vi "Build Menu from Graph.vi"(7 "Selection":i32, 10 "Items":T1[](array[typedef]), 11 "Menu":refnum<k9>) -> ()   [LabVIEW 2016, in "Better Search.lvlib"]
uses:
  Better Search.lvlib
  Data Types/Type Reflection Item.ctl
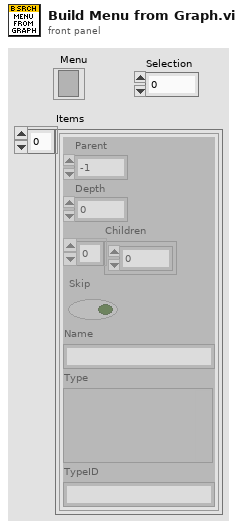
[diagram p1: front panel]
types:
  T1 = typedef "Better Search.lvlib/Type Reflection Item.ctl" = cluster{"Parent":i32, "Depth":i32, "Children":i32[], "Skip":bool, "Name":string, "Type":variant, "TypeID":string}
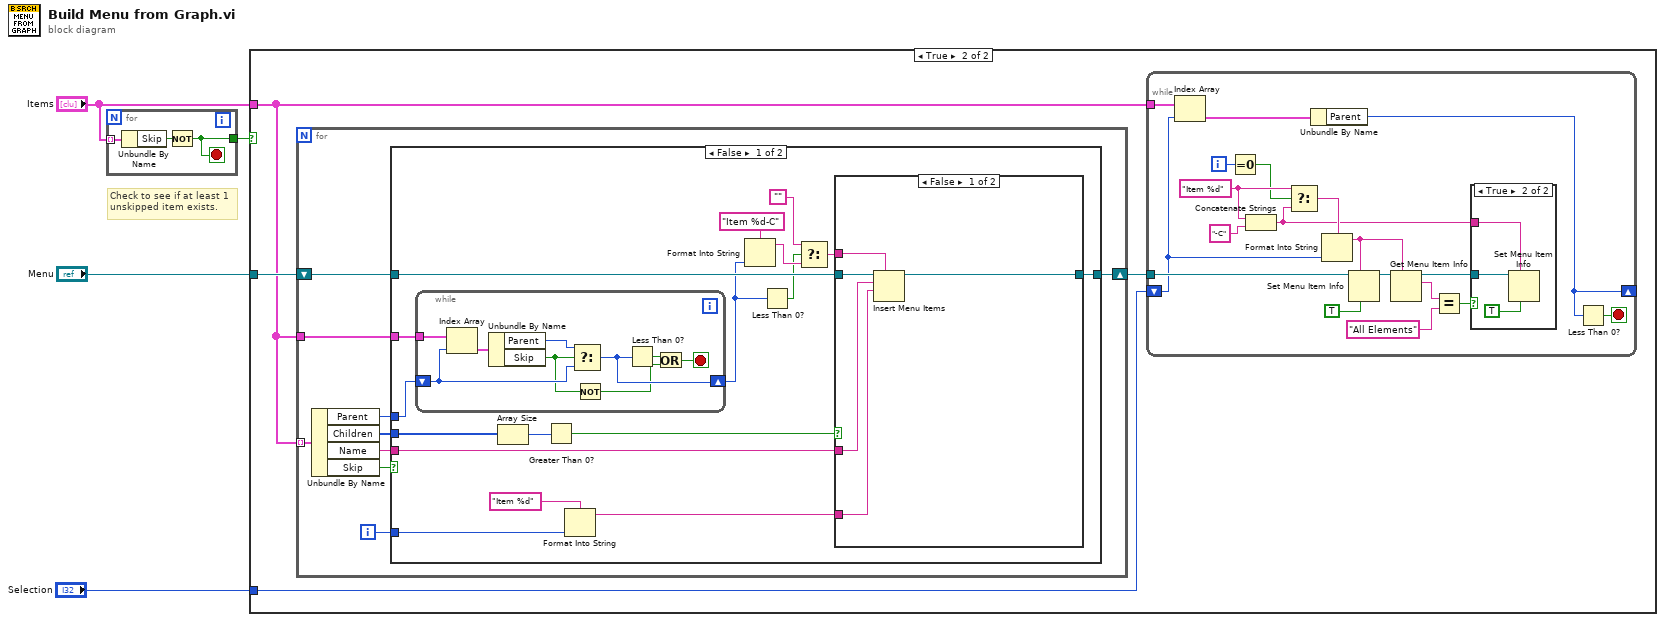
[diagram p0: block diagram]
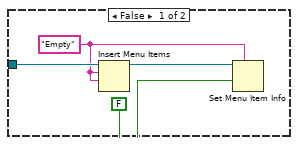
[diagram p2: hidden frame]
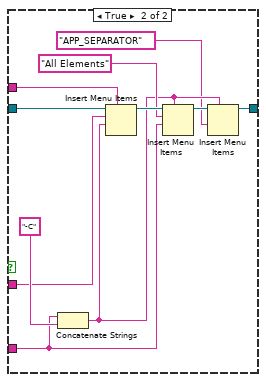
[diagram p3: hidden frame]
diagram:
  # "Check to see if at least 1 unskipped item exists."
  n1 = for {
    tunnel: "Items" -> [w7] mode=indexing
    tunnel: [w5] -> w1
    stop <- w5 stop-if-true
    n2 = Unbundle By Name(w7) -> ("Skip"=w6:bool)
    n3 = Not(x=w6) -> (.not. x?=w5:bool)
  }
  n4 = case shown="True" w1 {
    tunnel: "Items" -> [_ w12]
    tunnel: "Menu" -> [w11 w15]
    tunnel: "Selection" -> [_ w13]
    frame False {
      w9 = "Empty"
      n5 = Insert Menu Items(7:w9, 8:w9, 9:w11) -> (3:w10:refnum<k9>)  [unwired: 3 in, 2 out]
      n6 = Set Menu Item Info(7:w9, 9:FALSE ("enabled"), 11:w10) -> ()  [unwired: 4 in, 2 out]
    }
    frame True {
      n7 = for {
        tunnel: w12 -> [w24] mode=indexing
        shift-right: [w17] -> w14
        shift-left: w15 -> [w20]
        tunnel: w12 -> [w16]
        i -> [w19]
        n8 = Unbundle By Name(w24) -> ("Parent"=w18:i32, "Children"=w21:i32[], "Name"=w22:string, "Skip"=w23:bool)
        n9 = case shown="False" w23 {
          tunnel: w22 -> [w28 _]
          tunnel: w21 -> [w41 _]
          tunnel: w20 -> [w37 w67]
          tunnel: w19 -> [w39 _]
          tunnel: w18 -> [w26 _]
          tunnel: [w34 w67] -> w17
          tunnel: w16 -> [w27 _]
          frame False {
            n10 = while {
              tunnel: w27 -> [w50]
              shift-right: [w45] -> w25
              shift-left: w26 -> [w47]
              stop <- w42 stop-if-true
              n11 = Index Array(array=w50, index=w47) -> (element=w49:T1)
              n12 = Unbundle By Name(w49) -> ("Parent"=w48:i32, "Skip"=w46:bool)
              n13 = Select(t=w48, s=w46, f=w47) -> (s? t:f=w45:i32)
              n14 = Not(x=w46) -> (.not. x?=w43:bool)
              n15 = Less Than 0?(x=w45) -> (x < 0?=w44:bool)
              n16 = Or(x=w44, y=w43) -> (x .or. y?=w42:bool)
            }
            n17 = Array Size(array=w41) -> (size(s)=w40:i32)
            n18 = Greater Than 0?(x=w40) -> (x > 0?=w38:bool)
            n19 = Format Into String(format string="Item %d", w39) -> (resulting string=w36:string)  [unwired: 2 in, 1 out]
            n20 = Format Into String(format string="Item %d-C", w25) -> (resulting string=w33:string)  [unwired: 2 in, 1 out]
            n21 = Less Than 0?(x=w25) -> (x < 0?=w30:bool)
            n22 = Select(t="", s=w30, f=w33) -> (s? t:f=w32:string)
            n23 = case shown="False" w38 {
              tunnel: w37 -> [w55 w65]
              tunnel: w36 -> [w53 w56]
              tunnel: w28 -> [w52 w64]
              tunnel: w32 -> [w54 w57]
              tunnel: [w51 w58] -> w34
              frame False {
                n24 = Insert Menu Items(5:w54, 7:w53, 8:w52, 9:w55) -> (3:w51:refnum<k9>)  [unwired: 2 in, 2 out]
              }
              frame True {
                n25 = Concatenate Strings(w56, "-C" ("string")) -> (w60:string)
                n26 = Insert Menu Items(5:w57, 7:w60, 8:w64, 9:w65) -> (3:w63:refnum<k9>)  [unwired: 2 in, 2 out]
                n27 = Insert Menu Items(5:w60, 7:w56, 8:"All Elements", 9:w63) -> (3:w61:refnum<k9>)  [unwired: 2 in, 2 out]
                n28 = Insert Menu Items(5:w60, 7:"APP_SEPARATOR", 9:w61) -> (3:w58:refnum<k9>)  [unwired: 3 in, 2 out]
              }
            }
          }
          frame True {
          }
        }
      }
      n29 = while {
        tunnel: w14 -> [w85]
        shift-right: [w82] -> _
        shift-left: w13 -> [w81]
        tunnel: w12 -> [w84]
        i -> [w74]
        stop <- w86 stop-if-true
        w71 = "Item %d"
        n30 = Index Array(array=w84, index=w81) -> (element=w83:T1)
        n31 = Equal To 0?(x=w74) -> (x = 0?=w69:bool)
        n32 = Concatenate Strings(w71, "-C" ("string")) -> (w68:string)
        n33 = Select(t=w71, s=w69, f=w68) -> (s? t:f=w70:string)
        n34 = Unbundle By Name(w83) -> ("Parent"=w82:i32)
        n35 = Format Into String(format string=w70, w81) -> (resulting string=w75:string)  [unwired: 2 in, 1 out]
        n36 = Set Menu Item Info(6:TRUE ("checked"), 7:w75, 11:w85) -> (3:w79:refnum<k9>)  [unwired: 4 in, 1 out]
        n37 = Get Menu Item Info(7:w75, 11:w79) -> (2:w78:string, 3:w76:refnum<k9>)  [unwired: 1 in, 5 out]
        n38 = Equal?(x=w78, y="All Elements") -> (x = y?=w73:bool)
        n39 = case shown="True" w73 {
          tunnel: w76 -> [_ w89]
          tunnel: w68 -> [_ w87]
          frame False {
          }
          frame True {
            n40 = Set Menu Item Info(6:TRUE ("checked"), 7:w87, 11:w89) -> ()  [unwired: 4 in, 2 out]
          }
        }
        n41 = Less Than 0?(x=w82) -> (x < 0?=w86:bool)
      }
    }
  }
